vi "Angle_Calibration.vi"() -> ()   [LabVIEW 2010]
uses:
  Anemometry Sub Vis/Controls/User_Specific_mode.ctl
  Anemometry Sub Vis/Gen Trav/Trav_mode.ctl
panel:
  in  "Simulate/Run":T1
  in  "Datum Z":dbl=275.0
  in  "Probe Orientation":dbl=-10.0
  in  "Probe Radius":dbl=180.0
  in  "Datum Y":dbl
  in  "Datum X":dbl=3000.0
  out "Demanded X":dbl=2822.7346042952854
  out "Demanded Y":dbl=31.25667105836792
  # "+ve swings probe in +ve y direction"
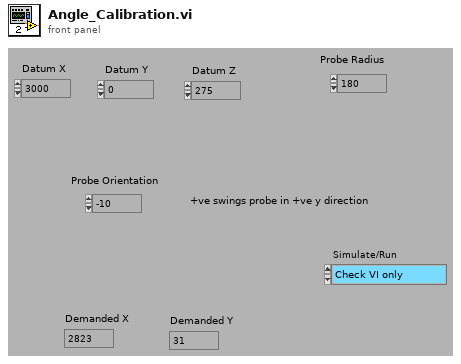
[diagram p1: front panel]
types:
  T1 = typedef "User_Specific_mode.ctl" = enum16{"Check VI only", "Run VI"}
  T2 = typedef "Trav_mode.ctl" = enum16{"Move traverse", "Read traverse position", "Teach Position"}
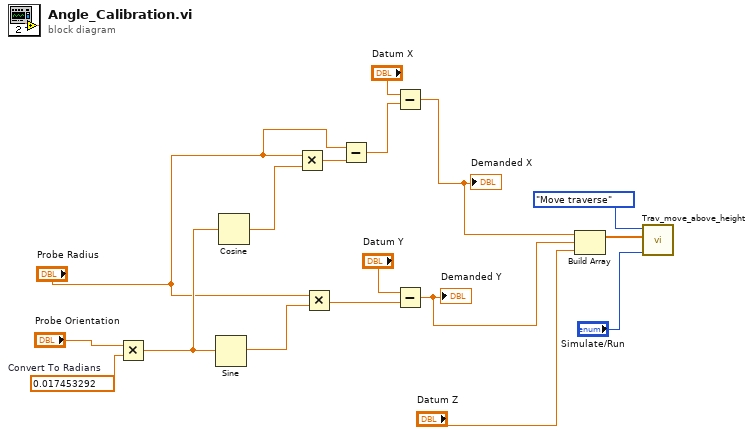
[diagram p0: block diagram]
diagram:
  w16 = 0.017453292  # Convert To Radians
  n1 = Multiply(x="Probe Orientation", y=w16) -> (x*y=w12:dbl)
  n2 = Sine(x=w12) -> (sin(x)=w15:dbl)
  n3 = Cosine(x=w12) -> (cos(x)=w11:dbl)
  n4 = Multiply(x="Probe Radius", y=w11) -> (x*y=w3:dbl)
  n5 = Multiply(x="Probe Radius", y=w15) -> (x*y=w13:dbl)
  n6 = Subtract(x="Probe Radius", y=w3) -> (x-y=w1:dbl)
  n7 = Subtract(x="Datum X", y=w1) -> (x-y=w9:dbl)
  "Demanded X" <- w9
  n8 = Subtract(x="Datum Y", y=w13) -> (x-y=w8:dbl)
  "Demanded Y" <- w8
  n9 = Build Array(w9, w8, "Datum Z") -> (w6:dbl[])
  n10 = call "Trav_move_above_height.vi"("Simulate/Run"="Simulate/Run", "New Position"=w6, "Mode"=Trav_mode."Move traverse") -> ()  [unwired: 7 in, 2 out]
